vi "GEA2 Filter Data.vi"(7 "Read ERD List":T1[](array[typedef]) {"ERD Number" format="%.0x"}, 8 "Error In":errorcluster, 11 "ERD Data Out in":T3[](array[typedef]) {"ERD Number" format="%.0x"}) -> (0 "Error Out":errorcluster, 2 "UnRead ERDs":i32, 3 "ERD Data Out out":T3[](array[typedef]) {"ERD Number" format="%.0x"})   [LabVIEW 2016]
uses:
  type defs/ERD Read Data Out.ctl
  type defs/ERD Read Data In.ctl
  type defs/Data Type.ctl
  library/GEA2_Toolkit.lvlib
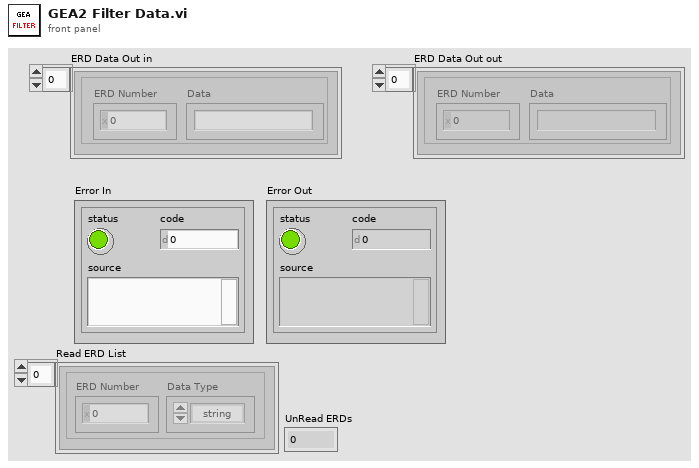
[diagram p1: front panel]
types:
  T1 = typedef "GEA2_Toolkit.lvlib/ERD Read Data In.ctl" = cluster{"ERD Number":u16, "Data Type":T2}
  T2 = typedef "GEA2_Toolkit.lvlib/Data Type.ctl" = enum16{"string", "boolean", "uint8_t", "uint16_t", "uint32_t", "uint64_t"}
  T3 = typedef "GEA2_Toolkit.lvlib/ERD Read Data Out.ctl" = cluster{"ERD Number":u16, "Data":string}
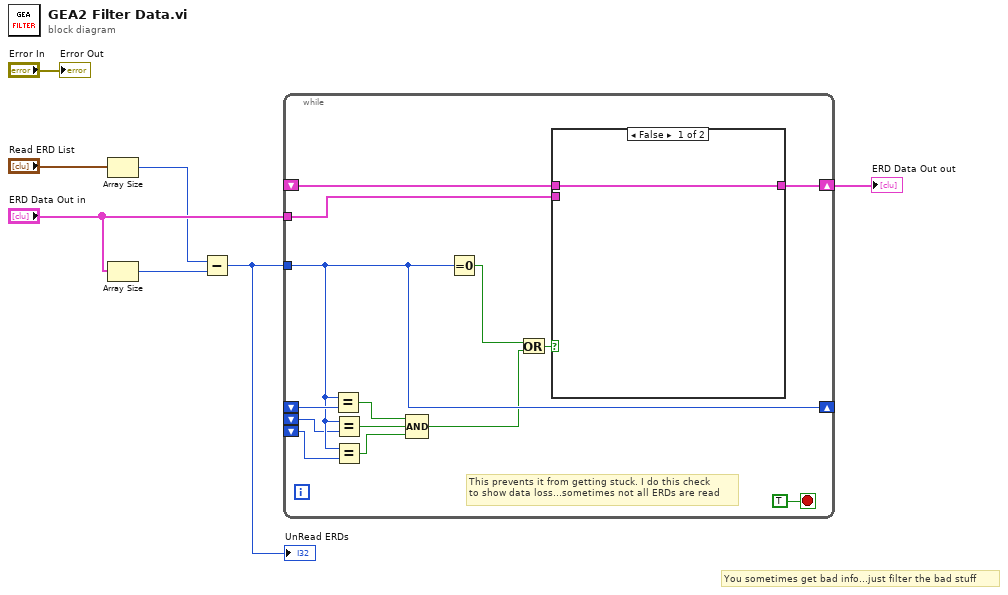
[diagram p0: block diagram]
diagram:
  # "You sometimes get bad info...just filter the bad stuff"
  n1 = Array Size(array="Read ERD List") -> (size(s)=w3:i32)
  n2 = Array Size(array="ERD Data Out in") -> (size(s)=w2:i32)
  n3 = Subtract(x=w3, y=w2) -> (x-y=w1:i32)
  "UnRead ERDs" <- w1
  n4 = while {
    shift-right: [w19] -> w7
    shift-left: _ -> [w18]
    tunnel: "ERD Data Out in" -> [w20]
    tunnel: w1 -> [w14]
    shift-right: [w14] -> _
    shift-left: _ -> [w15]
    shift-left: _ -> [w13]
    shift-left: _ -> [w12]
    stop <- TRUE stop-if-true
    # "This prevents it from getting stuck. I do this check\nto show data loss...sometimes not all ERDs are read"
    n5 = Equal?(x=w14, y=w15) -> (x = y?=w11:bool)
    n6 = Equal?(x=w14, y=w13) -> (x = y?=w10:bool)
    n7 = Equal?(x=w14, y=w12) -> (x = y?=w9:bool)
    n8 = Compound Arithmetic op=AND(w11, w10, w9) -> (w8:bool)
    n9 = Equal To 0?(x=w14) -> (x = 0?=w17:bool)
    n10 = Or(x=w17, y=w8) -> (x .or. y?=w16:bool)
    n11 = case shown="False" w16 {
      tunnel: w20 -> [_ w23]
      tunnel: [w22 w23] -> w19
      tunnel: w18 -> [w22 _]
      frame False {
      }
      frame True {
      }
    }
  }
  "ERD Data Out out" <- w7
  "Error Out" <- "Error In"
